vi "switch_post.vi"(7 "LabVIEW Web Service Request":refnum<class "Web Request.lvclass">) -> ()   [LabVIEW 2014]
uses:
  <vilib>/wsapi/Web Request.lvclass
  DataManager/StateStore/Controls/DataFunction.ctl
panel:
  out "timing post SW 2":u32
  out "error out":errorcluster
  # "Use the Web Service Request input terminal to call the VIs on the Web Services palette. Do not remove it from the connector pane unless you don't need access to the palette."
  # "Each additional control wired to the connector pane will be available as an input in the URL. To include an indicator in terminal-mode output (the default setting), it must also be wired to the connector pane."
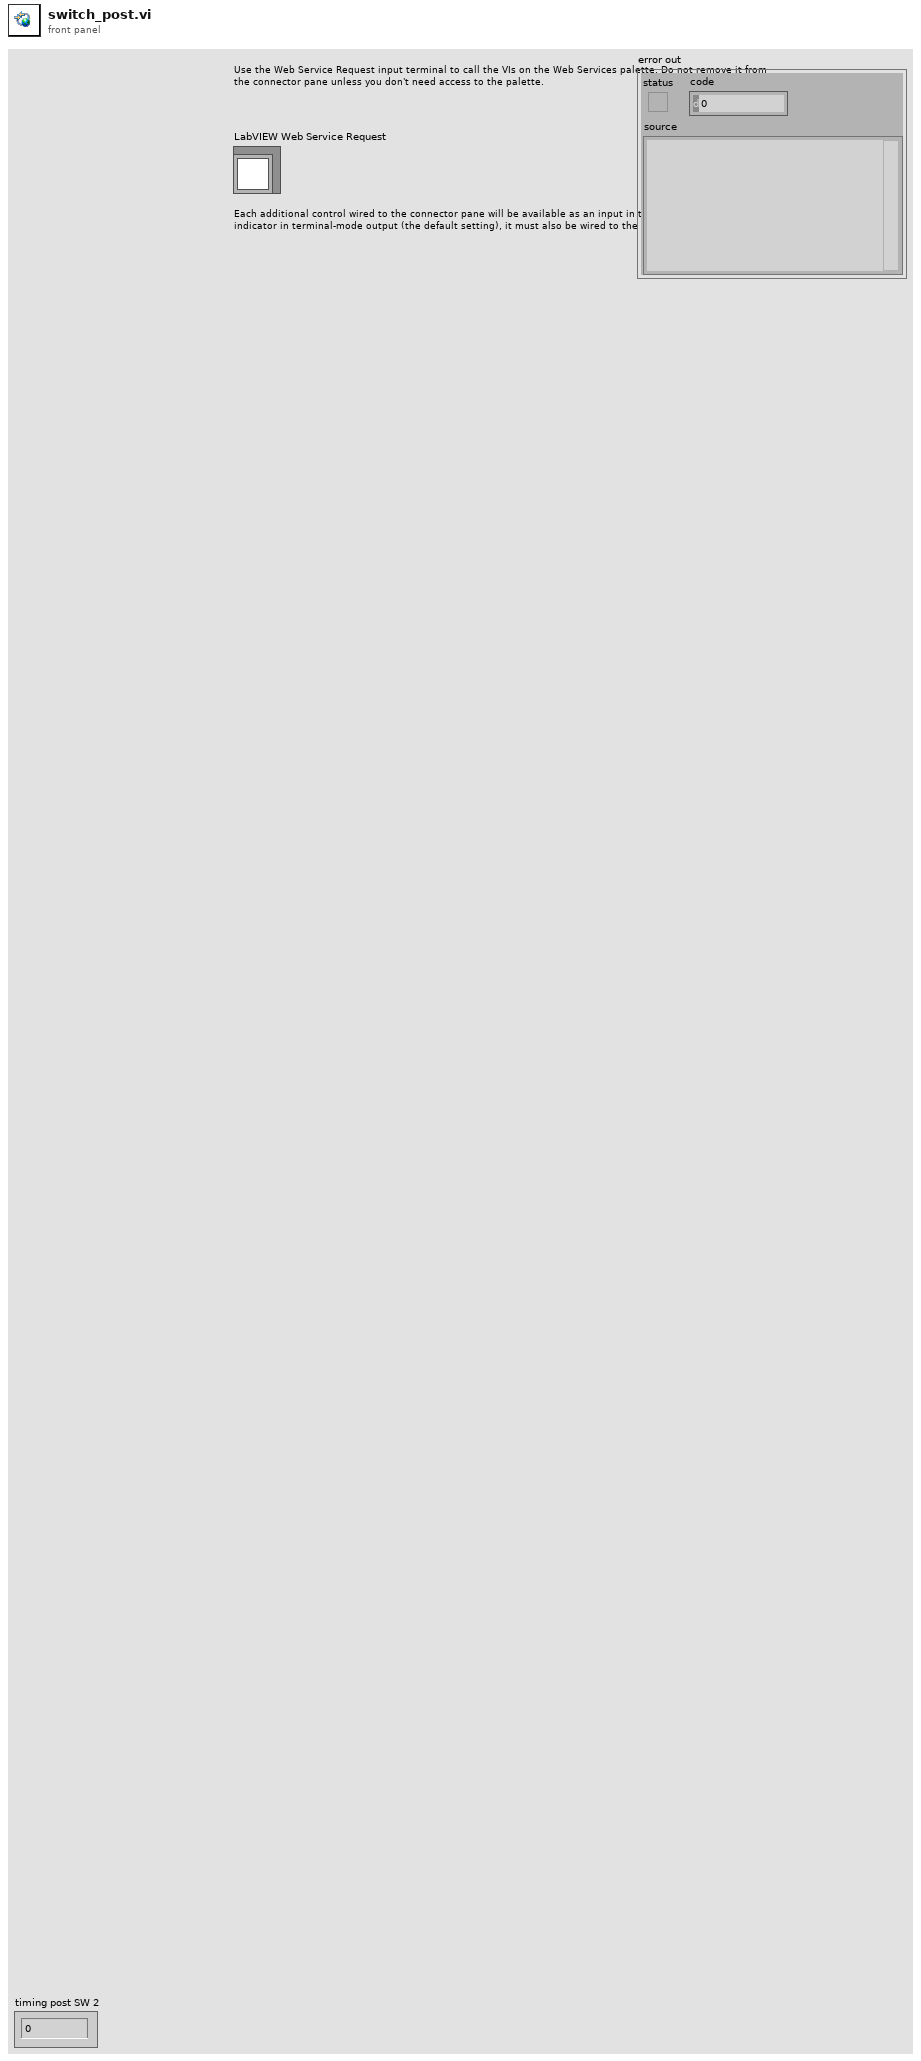
[diagram p1: front panel]
types:
  T1 = cluster{"switch_posit":cluster{"x":dbl, "y":dbl, "z":dbl}, "manual":bool}
  T2 = typedef "DataFunction.ctl" = enum16{"Initialise", "Release", "Get Data", "Set Data", "Preview Data"}
  T3 = typedef "CData Core Control.ctl" = cluster{"train_data_array":cluster{"uuid":string, "int":i32, "posit_array":cluster{"x":dbl, "y":dbl, "z":dbl}[]}[], "train_control_array":cluster{"uuid":string, "throttle":dbl, "brake":dbl, "horn":dbl, "wait":dbl, "name":string, "mode":string, "dest":string}[], "switch_data_array":cluster{"switch_posit":cluster{"x":dbl, "y":dbl, "z":dbl}, "manual":bool}[], "switch_control_array":cluster{"switch_posit":cluster{"x":dbl, "y":dbl, "z":dbl}, "switch":bool, "invert":bool, "wait":dbl}[]}
  T4 = cluster{"switch_posit":cluster{"x":dbl, "y":dbl, "z":dbl}, "manual":bool}[]
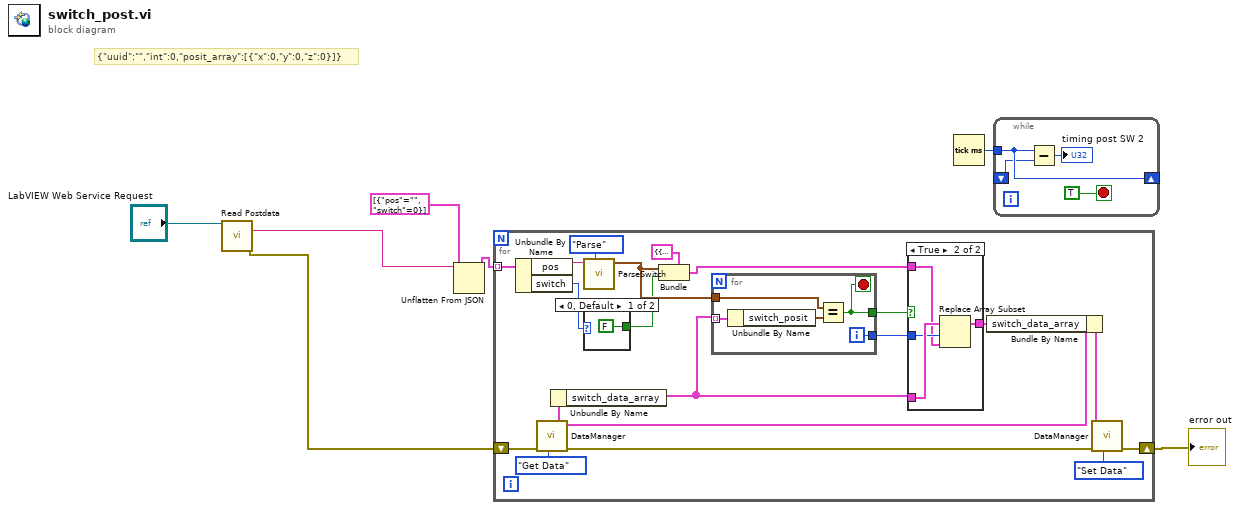
[diagram p0: block diagram]
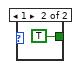
[diagram p2: hidden frame]
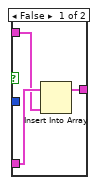
[diagram p3: hidden frame]
diagram:
  # "{\"uuid\":\"\",\"int\":0,\"posit_array\":[{\"x\":0,\"y\":0,\"z\":0}]}"
  n1 = call <vilib>:"Read Postdata.vi"("LabVIEW Web Service Request"="LabVIEW Web Service Request") -> ("postdata"=w3:string, "error out"=w2:errorcluster)  [unwired: 12 in, 1 out]
  n2 = Unflatten From JSON(JSON string=w3, type and defaults=cluster{"pos":string, "switch":i32}[] [{"pos"="", "switch"=0}]) -> (value=w4:cluster{"pos":string, "switch":i32}[])  [unwired: 5 in, 1 out]
  n3 = for {
    shift-right: [w19] -> w1
    shift-left: w2 -> [w17]
    tunnel: w4 -> [w16] mode=indexing
    n4 = Unbundle By Name(w16) -> ("pos"=w15:string, "switch"=w9:i32)
    n5 = call "DataManager.vi"("DataFunction"=DataFunction."Get Data", "error in (no error)"=w17) -> ("error out"=w18:errorcluster, "CData Out"=w20:T3)  [unwired: 8 in]
    n6 = Unbundle By Name(w20) -> ("switch_data_array"=w14:T4)
    n7 = call "ParseSwitch.vi"("Enum"=enum16{"Parse", "Convert to string"}."Parse", "String"=w15) -> ("output cluster"=w12:cluster{"x":dbl, "y":dbl, "z":dbl})  [unwired: 8 in, 1 out]
    n8 = case shown="0, Default" w9 {
      tunnel: [FALSE ("manual") TRUE ("manual")] -> w8
      frame 0, Default {
      }
      frame 1 {
      }
    }
    n9 = Bundle(cluster=T1 {"switch_posit"={"x"=0.0, "y"=0.0, "z"=0.0}, "manual"=FALSE} ("new element/subarray"), "switch_posit"=w12, "manual"=w8) -> (w11:T1)
    n10 = for {
      tunnel: w14 -> [w40] mode=indexing
      tunnel: [w38] -> w23
      tunnel: [w37] -> w22
      tunnel: w12 -> [w36]
      i -> [w37]
      stop <- w38 stop-if-true
      n11 = Unbundle By Name(w40) -> ("switch_posit"=w39:cluster{"x":dbl, "y":dbl, "z":dbl})
      n12 = Equal?(x=w36, y=w39) -> (x = y?=w38:bool)
    }
    n13 = case shown="True" w23 {
      tunnel: w22 -> [_ w34]
      tunnel: w14 -> [w31 w35]
      tunnel: w11 -> [w30 w32]
      tunnel: [w29 w33] -> w21
      frame False {
        n14 = Insert Into Array(array=w31, new element=w30) -> (w29:T4)  [unwired: 1 in]
      }
      frame True {
        n15 = Replace Array Subset(array=w35, new element=w32, index=w34) -> (w33:T4)
      }
    }
    n16 = Bundle By Name(cluster=w20, "switch_data_array"=w21) -> (w24:T3)
    n17 = call "DataManager.vi"("DataFunction"=DataFunction."Set Data", "error in (no error)"=w18, "CData In"=w24) -> ("error out"=w19:errorcluster)  [unwired: 7 in, 1 out]
  }
  "error out" <- w1
  n18 = Tick Count (ms)() -> (millisecond timer value=w6:u32)
  n19 = while {
    tunnel: w6 -> [w44]
    shift-right: [w44] -> _
    shift-left: _ -> [w43]
    stop <- TRUE stop-if-true
    n20 = Subtract(x=w44, y=w43) -> (x-y=→"timing post SW 2":u32)
  }
